vi "GenesysPS.Initialize.vi"(0 "i ref in":refnum<vi>, 5 "error in (no error)":errorcluster) -> (14 "i ref out":refnum<vi>, 19 "error out":errorcluster)   [LabVIEW 2014, in "GenesysPS.lvlib"]
doc: "Initializes the connection and the PS.\n\nLicense Agreement for this software:\n\nCopyright (C)\nGesellschaft für Schwerionenforschung, GSI\nPlanckstr. 1\n64291 Darmstadt\nGermany\n\nContact: D.Beck@gsi.de \n\nThis program is free software; you can redistribute it and/or modify it under the terms of the GNU General Public License as published by the Free Software Foundation; either version 2 of the license, or (at your option) any later version.\n\nThis program is distributed in the hope that it will be useful, but WITHOUT ANY WARRANTY; without even the implied warranty of MERCHANTABILITY or FITNESS FOR A PARTICULAR PURPOSE. See the GNU General License for more details (http://www.gnu.org).\n\nGesellschaft für Schwerionenforschung, GSI\nPlanckstr. 1, 64291 Darmstadt, Germany\nFor all questions and ideas contact: M.Richter@gsi.de, H.Brand@gsi.de or D.Beck@gsi.de.\nLast update: 17-JUN-2004"
uses:
  GenesysPS.lvlib
  instr.lib/GENser/GENserDriver.lvlib
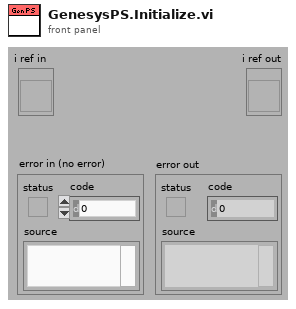
[diagram p1: front panel]
types:
  T1 = typedef "GenesysPS.lvlib/GenesysPS.i attribute.ctl" = cluster{"VISA name/ Heizinger":refnum<visa-resource-name>, "GEN Addr":i32, "WithTempInt?":bool, "TempLimit":dbl, "TemperatureID":i32, "Temp queue":refnum<queue>}
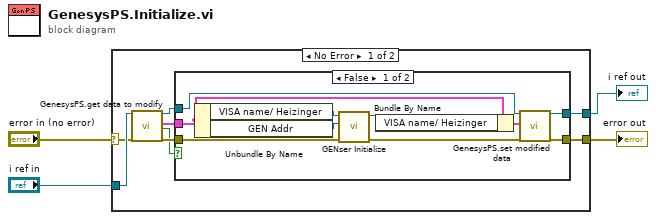
[diagram p0: block diagram]
diagram:
  n1 = case shown="No Error" "error in (no error)" {
    selector: "error in (no error)" -> [w11 w26]
    tunnel: [w9 w26] -> w4
    tunnel: [w7 w25] -> w2
    tunnel: "i ref in" -> [w12 w25]
    frame No Error {
      n2 = call "GenesysPS.get data to modify.vi"("i ref in"=w12, "error in (no error)"=w11) -> ("i ref out"=w8:refnum<vi>, "i attribute"=w6:T1, "timed out"=w5:bool, "error out"=w10:errorcluster)  [unwired: 14 in]
      n3 = case shown="False" w5 {
        tunnel: w10 -> [w20 w23]
        tunnel: [w18 w23] -> w9
        tunnel: w8 -> [w17 w24]
        tunnel: [w16 w24] -> w7
        tunnel: w6 -> [w14 _]
        frame False {
          n4 = Unbundle By Name(w14) -> ("VISA name/ Heizinger"=w22:refnum<visa-resource-name>, "GEN Addr"=w21:i32)
          n5 = call "GENser Initialize.vi"("error in (no error)"=w20, "GEN Addr"=w21, "VISA name"=w22) -> ("error out"=w19:errorcluster, "VISA out"=w13:refnum<visa-resource-name>)  [unwired: 7 in]
          n6 = Bundle By Name(cluster=w14, "VISA name/ Heizinger"=w13) -> (w15:T1)
          n7 = call "GenesysPS.set modified data.vi"("i ref in"=w17, "i attribute"=w15, "error in (no error)"=w19) -> ("i ref out"=w16:refnum<vi>, "error out"=w18:errorcluster)  [unwired: 15 in]
        }
        frame True {
        }
      }
    }
    frame Error {
    }
  }
  "i ref out" <- w2
  "error out" <- w4
